vi "tm_addnewregion_40.vi"(8 "error in (no error)":errorcluster, 10 "Sub Region":T1, 11 "Handle in":u32) -> (0 "error out":errorcluster, 3 "Handle out":u32)   [LabVIEW 2011]
uses:
  tmcamcon.dll
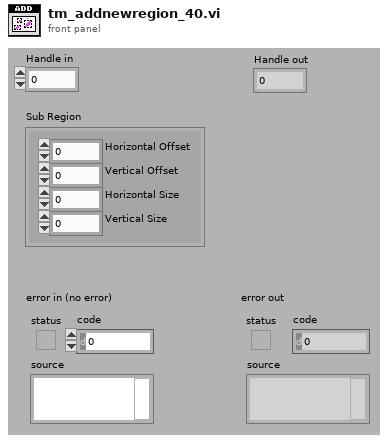
[diagram p1: front panel]
types:
  T1 = cluster{"Horizontal Offset":i32, "Vertical Offset":i32, "Horizontal Size":i32, "Vertical Size":i32}
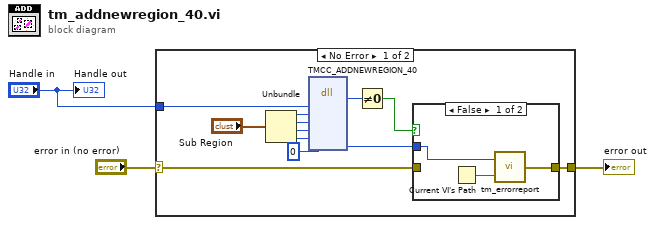
[diagram p0: block diagram]
diagram:
  n1 = case shown="No Error" "error in (no error)" {
    selector: "error in (no error)" -> [w9 w20]
    tunnel: [w6 w20] -> w2
    tunnel: "Handle in" -> [w10 _]
    frame No Error {
      n2 = Unbundle("Sub Region") -> ("Horizontal Offset"=w14:i32, "Vertical Offset"=w13:i32, "Horizontal Size"=w12:i32, "Vertical Size"=w11:i32)
      n3 = dll-call lib="tmcamcon.dll" fn="TMCC_ADDNEWREGION_40"("index"=w10, "left"=w14, "top"=w13, "right"=w12, "bottom"=w11, "Erval"=0) -> ("return type"=w15:u32, "Erval"=w8:i32)  [unwired: 8 in, 2 out]
      n4 = Not Equal To 0?(x=w15) -> (x != 0?=w7:bool)
      n5 = case shown="False" w7 {
        tunnel: w9 -> [_ w19]
        tunnel: [w17 w19] -> w6
        tunnel: w8 -> [w16 _]
        frame False {
          n6 = Current VI's Path() -> (path=w18:path)
          n7 = call <userlib>:"tm_errorreport.vi"("Source"=w18, "Error"=w16) -> ("error out"=w17:errorcluster)
        }
        frame True {
        }
      }
    }
    frame Error {
    }
  }
  "error out" <- w2
  "Handle out" <- "Handle in"
